vi "Test.vi"() -> ()   [LabVIEW 2009, in "OccupancyMap.lvclass"]
uses:
  OccupancyMap.lvclass
  parameters.ctl
  Rectangle/Rectangle.lvclass
panel:
  out "Map":picture
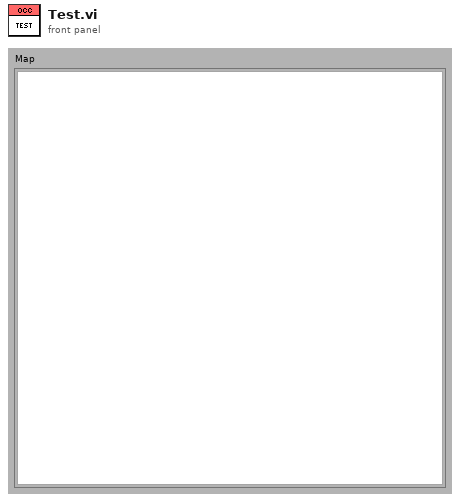
[diagram p1: front panel]
types:
  T1 = cluster{"left":i16, "top":i16, "right":i16, "bottom":i16}
  T2 = cluster{"Width":i16, "Style":enum32{"Solid", "Dash", "Dot", "DashDot", "DashDotDot"}}
  T3 = cluster{"Left":dbl, "Right":dbl, "Top":dbl, "Bottom":dbl}
  T4 = cluster{"Width":u16, "Style":enum32{"Solid", "Dash", "Dot", "DashDot", "DashDotDot"}}
  T5 = typedef "OccupancyMap.lvclass/parameters.ctl" = cluster{"MapResolution":cluster{"resX":dbl, "resY":dbl}, "StartLocation":cluster{"X":dbl, "Y":dbl}, "Goal":cluster{"X":dbl, "Y":dbl}, "MapBoundaries":cluster{"Left":dbl, "Right":dbl, "Top":dbl, "Bottom":dbl}}
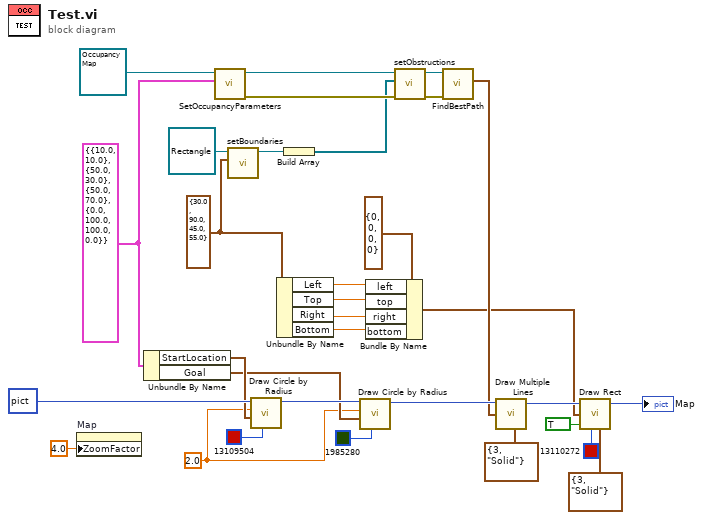
[diagram p0: block diagram]
diagram:
  w6 = T3 {"Left"=30.0, "Right"=90.0, "Top"=45.0, "Bottom"=55.0} ("Boundaries")
  w21 = sgl 2.0 ("Zoom Factor")
  w30 = T5 {"MapResolution"={"resX"=10.0, "resY"=10.0}, "StartLocation"={"X"=50.0, "Y"=30.0}, "Goal"={"X"=50.0, "Y"=70.0}, "MapBoundaries"={"Left"=0.0, "Right"=100.0, "Top"=100.0, "Bottom"=0.0}} ("Parameters")
  n1 = property on="Map" class="Pict"("ZoomFactor"=sgl 4.0 ("Zoom Factor")) -> ()  [unwired: 2 in, 2 out]
  n2 = Unbundle By Name(w30) -> ("StartLocation"=w29:cluster{"X":dbl, "Y":dbl}, "Goal"=w27:cluster{"X":dbl, "Y":dbl})
  n3 = call "SetOccupancyParameters.vi"("Parameters"=w30, "OccupancyMap in"=refnum<class "OccupancyMap.lvclass"> refnum) -> ("error out"=w17:errorcluster, "OccupancyMap out"=w18:refnum<class "OccupancyMap.lvclass">)  [unwired: 8 in]
  n4 = call "setBoundaries.vi"("Boundaries"=w6, "Rectangle in"=refnum<class "Rectangle.lvclass"> refnum ("Rectangle.lvclass")) -> ("Rectangle out"=w11:refnum<class "Rectangle.lvclass">)  [unwired: 8 in, 1 out]
  n5 = call <vilib>:"Draw Circle by Radius.vi"("color(black)"=u32 13109504, "pixel center"=w29, "radius"=w21, "picture"=picture data[5B] ("2D Picture")) -> ("new picture"=w28:picture)  [unwired: 7 in]
  n6 = Unbundle By Name(w6) -> ("Left"=w5:dbl, "Top"=w4:dbl, "Right"=w3:dbl, "Bottom"=w2:dbl)
  n7 = Build Array(w11) -> (w16:refnum<class "Rectangle.lvclass">[])
  n8 = call <vilib>:"Draw Circle by Radius.vi"("color(black)"=u32 1985280, "pixel center"=w27, "radius"=w21, "picture"=w28) -> ("new picture"=w24:picture)  [unwired: 7 in]
  n9 = Bundle By Name(cluster=T1 {"left"=0, "top"=0, "right"=0, "bottom"=0} ("rect"), "left"=w5, "top"=w4, "right"=w3, "bottom"=w2) -> (w1:T1)
  n10 = call "setObstructions.vi"("error in (no error)"=w17, "Obstructions"=w16, "OccupancyMap in"=w18) -> ("error out"=w20:errorcluster, "OccupancyMap out"=w19:refnum<class "OccupancyMap.lvclass">)  [unwired: 7 in]
  n11 = call "FindBestPath.vi"("error in (no error)"=w20, "OccupancyMap in"=w19) -> ("path"=w23:cluster{"X":dbl, "Y":dbl}[])  [unwired: 6 in, 3 out]
  n12 = call <vilib>:"Draw Multiple Lines.vi"("picture"=w24, "line endpoints"=w23, "pen"=T4 {"Width"=3, "Style"=enum."Solid"}) -> ("new picture"=w15:picture)  [unwired: 6 in]
  n13 = call <vilib>:"Draw Rect.vi"("picture"=w15, "rect"=w1, "fill?(F)"=TRUE, "color(black)"=u32 13110272, "pen"=T2 {"Width"=3, "Style"=enum."Solid"}) -> ("new picture"=→"Map":picture)  [unwired: 4 in]
